vi "FET_Test_Config_4275A.vi"(7 "LowCapMode?":bool, 8 "error in":errorcluster, 9 "Test Mode":bool=TRUE, 10 "Device Type":string, 11 "FET Test Configuration":string) -> (0 "error out":errorcluster)   [LabVIEW 2020]
uses:
  Global 1.vi
panel:
  in  "Keystate":string
  # "True = Normal Mode\nFalse = Hi-Res"
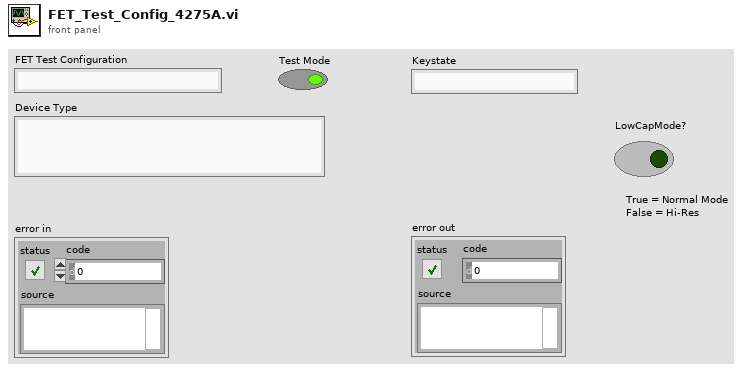
[diagram p1: front panel]
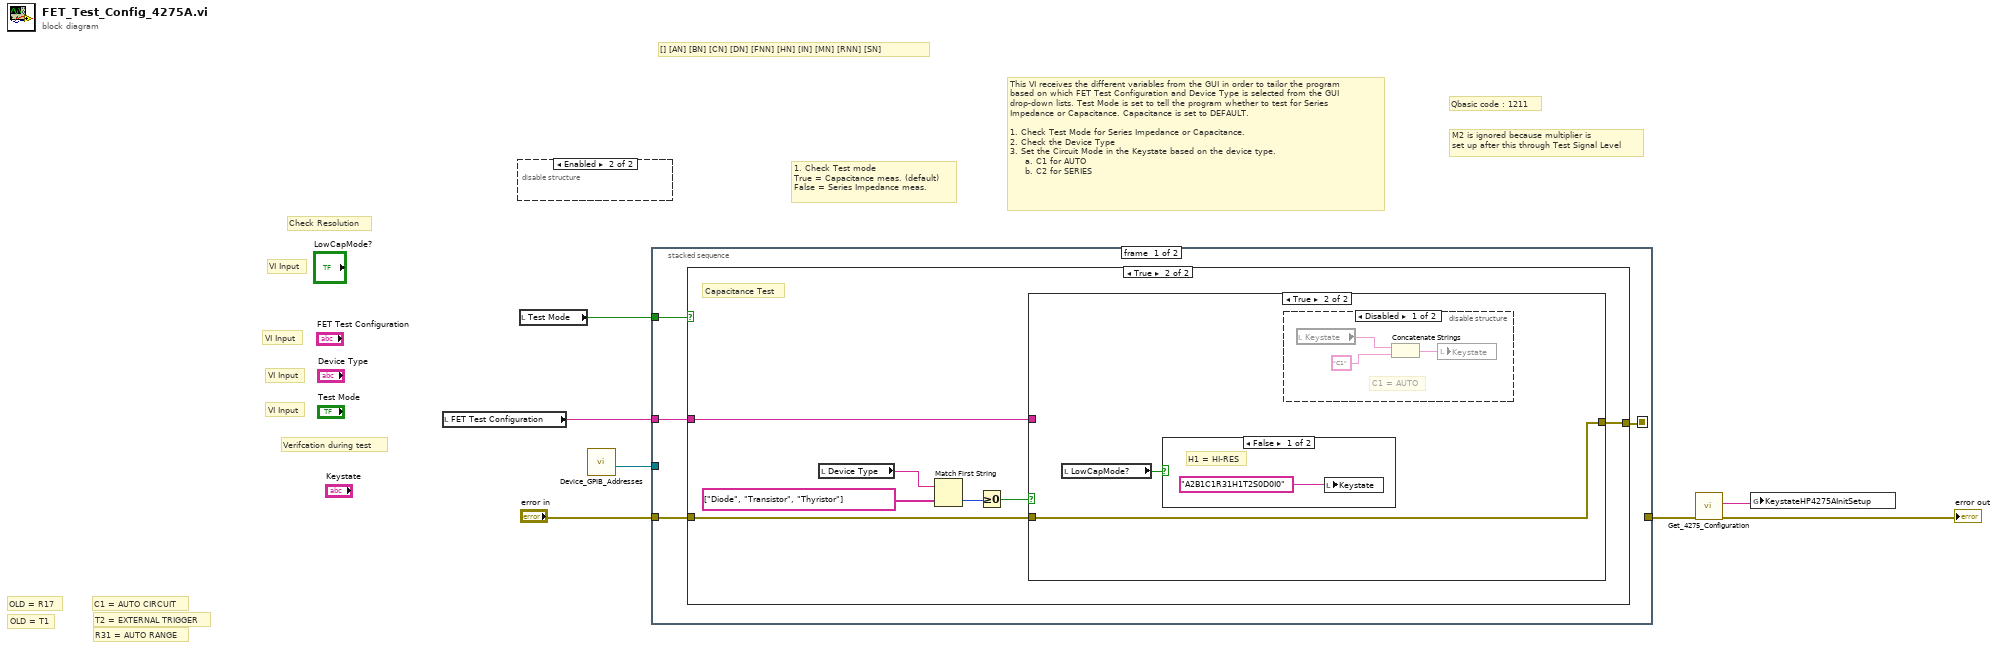
[diagram p0: block diagram]
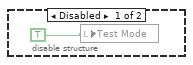
[diagram p2: hidden frame]
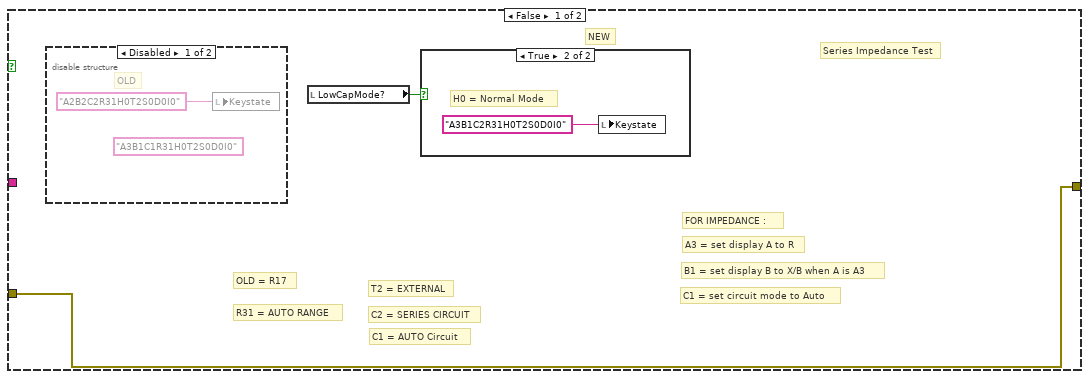
[diagram p3: hidden frame]
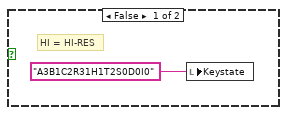
[diagram p4: hidden frame]
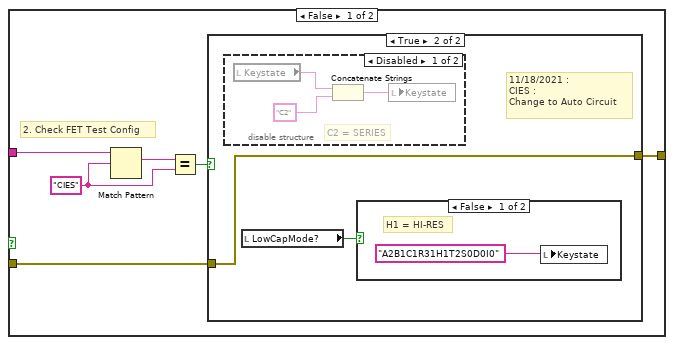
[diagram p6: hidden frame]
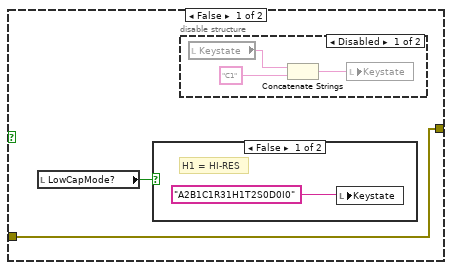
[diagram p7: hidden frame]
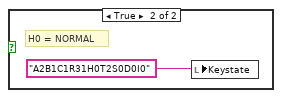
[diagram p8: hidden frame]
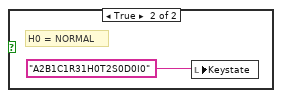
[diagram p10: hidden frame]
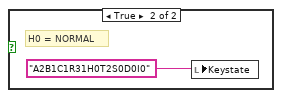
[diagram p12: hidden frame]
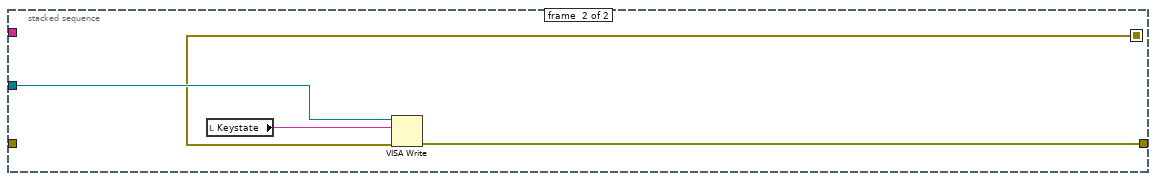
[diagram p14: hidden frame]
diagram:
  # "T2 = EXTERNAL TRIGGER"
  # "OLD = T1"
  # "C1 = AUTO CIRCUIT"
  # "R31 = AUTO RANGE"
  # "OLD = R17"
  # "Qbasic code : 1211"
  # "M2 is ignored because multiplier is\nset up after this through Test Signal Level"
  # "Check Resolution"
  # "VI Input"
  # "[] [AN] [BN] [CN] [DN] [FNN] [HN] [IN] [MN] [RNN] [SN]"
  # "This VI receives the different variables from the GUI in order to tailor the program\nbased on which FET Test Configuration and Device Type is selected from the GUI\ndrop-down lists. Test Mode is set to tell the program whether to test for Series\nImpedance or Capacitance. Capacitance is set to DEFAULT. \n\n1. Check Test Mode for Series Impedance or Capacitance.\n2. Check the Device Type\n3. Set the Circuit Mode in the Keystate based on the device type.\n     a. C1 for AUTO\n     b. C2 for SERIES"
  # "Verifcation during test"
  # "1. Check Test mode\nTrue = Capacitance meas. (default)\nFalse = Series Impedance meas."
  # "VI Input"
  # "VI Input"
  # "VI Input"
  n1 = local read "FET Test Configuration"() -> (w6:string)
  n2 = disable-structure shown="Enabled" {
    frame Disabled {
      n3 = local write "Test Mode"(TRUE ("Test Mode")) -> ()
    }
    frame Enabled {
    }
  }
  n4 = local read "Test Mode"() -> (w7:bool)
  n5 = call "Device_GPIB_Addresses.vi"() -> ("HP 4275A Address"=w4:refnum<visa-resource-name>)  [unwired: 9 in, 2 out]
  n6 = stacked-sequence {
    seq-local: [w9 _] -> [_ w52]
    tunnel: w7 -> [w12 _]
    tunnel: w6 -> [w11 _]
    tunnel: "error in" -> [w10 _]
    tunnel: [_ w53] -> w3
    tunnel: w4 -> [_ w54]
    frame #0 {
      n7 = case shown="True" w12 {
        tunnel: w11 -> [_ w20]
        tunnel: w10 -> [w13 w18]
        tunnel: [w13 w19] -> w9
        frame False {
          # "C1 = set circuit mode to Auto"
          # "NEW"
          # "C1 = AUTO Circuit"
          # "B1 = set display B to X/B when A is A3"
          # "A3 = set display A to R"
          # "FOR IMPEDANCE :"
          # "C2 = SERIES CIRCUIT"
          # "T2 = EXTERNAL"
          # "R31 = AUTO RANGE"
          # "OLD = R17"
          # "Series Impedance Test"
          n8 = disable-structure shown="Disabled" {
            frame Disabled {
              (unwired) "A3B1C1R31H0T2S0D0I0" ("Keystate")
              # "OLD"
              n9 = local write "Keystate"("A2B2C2R31H0T2S0D0I0" ("Keystate")) -> ()
            }
            frame Enabled {
            }
          }
          n10 = local read "LowCapMode?"() -> (w14:bool)
          n11 = case shown="True" w14 {
            frame False {
              # "HI = HI-RES"
              n12 = local write "Keystate"("A3B1C2R31H1T2S0D0I0" ("Keystate")) -> ()
            }
            frame True {
              # "H0 = Normal Mode"
              n13 = local write "Keystate"("A3B1C2R31H0T2S0D0I0" ("Keystate")) -> ()
            }
          }
        }
        frame True {
          # "Capacitance Test"
          n14 = local read "Device Type"() -> (w24:string)
          n15 = Match First String(2:string[] ["Diode", "Transistor", "Thyristor"] ("string array"), 3:w24) -> (0:w22:i32)  [unwired: 1 out]
          n16 = Greater Or Equal To 0?(x=w22) -> (x >= 0?=w21:bool)
          n17 = case shown="True" w21 {
            tunnel: w20 -> [w27 _]
            tunnel: [w26 w45] -> w19
            tunnel: w18 -> [w25 w45]
            frame False {
              w28 = "CIES" ("regular expression")
              # "2. Check FET Test Config"
              n18 = Match Pattern(string=w27, regular expression=w28) -> (match substring=w29:string)  [unwired: 1 in, 3 out]
              n19 = Equal?(x=w29, y=w28) -> (x = y?=w30:bool)
              n20 = case shown="True" w30 {
                tunnel: [w31 w38] -> w26
                tunnel: w25 -> [w31 w38]
                frame False {
                  n21 = local read "LowCapMode?"() -> (w32:bool)
                  n22 = case shown="False" w32 {
                    frame False {
                      # "H1 = HI-RES"
                      n23 = local write "Keystate"("A2B1C1R31H1T2S0D0I0" ("Keystate")) -> ()
                    }
                    frame True {
                      # "H0 = NORMAL"
                      n24 = local write "Keystate"("A2B1C1R31H0T2S0D0I0" ("Keystate")) -> ()
                    }
                  }
                  n25 = disable-structure shown="Disabled" {
                    frame Disabled {
                      n26 = local read "Keystate"() -> (w36:string)
                      n27 = Concatenate Strings(w36, "C1" ("string")) -> (w37:string)
                      n28 = local write "Keystate"(w37) -> ()
                    }
                    frame Enabled {
                    }
                  }
                }
                frame True {
                  # "11/18/2021 :\nCIES :\nChange to Auto Circuit"
                  n29 = disable-structure shown="Disabled" {
                    frame Disabled {
                      # "C2 = SERIES"
                      n30 = local read "Keystate"() -> (w44:string)
                      n31 = Concatenate Strings(w44, "C2" ("wrt")) -> (w42:string)
                      n32 = local write "Keystate"(w42) -> ()
                    }
                    frame Enabled {
                    }
                  }
                  n33 = local read "LowCapMode?"() -> (w39:bool)
                  n34 = case shown="False" w39 {
                    frame False {
                      # "H1 = HI-RES"
                      n35 = local write "Keystate"("A2B1C1R31H1T2S0D0I0" ("Keystate")) -> ()
                    }
                    frame True {
                      # "H0 = NORMAL"
                      n36 = local write "Keystate"("A2B1C1R31H0T2S0D0I0" ("Keystate")) -> ()
                    }
                  }
                }
              }
            }
            frame True {
              n37 = local read "LowCapMode?"() -> (w46:bool)
              n38 = case shown="False" w46 {
                frame False {
                  # "H1 = HI-RES"
                  n39 = local write "Keystate"("A2B1C1R31H1T2S0D0I0" ("Keystate")) -> ()
                }
                frame True {
                  # "H0 = NORMAL"
                  n40 = local write "Keystate"("A2B1C1R31H0T2S0D0I0" ("Keystate")) -> ()
                }
              }
              n41 = disable-structure shown="Disabled" {
                frame Disabled {
                  # "C1 = AUTO"
                  n42 = local read "Keystate"() -> (w50:string)
                  n43 = Concatenate Strings(w50, "C1" ("wrt")) -> (w51:string)
                  n44 = local write "Keystate"(w51) -> ()
                }
                frame Enabled {
                }
              }
            }
          }
        }
      }
    }
    frame #1 {
      n45 = local read "Keystate"() -> (w55:string)
      n46 = VISA Write(VISA resource name=w54, write buffer=w55, error in (no error)=w52) -> (error out=w53:errorcluster)  [unwired: 2 out]
    }
  }
  n47 = call "Get_4275_Configuration.vi"("error in"=w3) -> ("error out"=→"error out":errorcluster, "Keystate"=w1:string)  [unwired: 9 in]
  n48 = global write "Global 1.vi" "KeystateHP4275AInitSetup"(w1) -> ()
